vi "DisconnectionRequest.vi"(8 "AuthKey":string, 10 "Server Port":i32, 11 "Server IP":string) -> ()   [LabVIEW 2016]
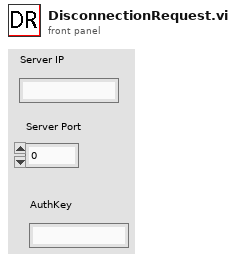
[diagram p1: front panel]
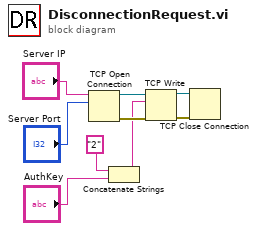
[diagram p0: block diagram]
diagram:
  n1 = TCP Open Connection(address="Server IP", remote port or service name="Server Port") -> (connection ID=w6:refnum<k5>, error out=w7:errorcluster)  [unwired: 3 in]
  n2 = Concatenate Strings("2", "AuthKey") -> (w3:string)
  n3 = TCP Write(connection ID=w6, data in=w3, error in (no error)=w7) -> (connection ID out=w2:refnum<k5>, error out=w1:errorcluster)  [unwired: 1 in, 1 out]
  n4 = TCP Close Connection(connection ID=w2, error in (no error)=w1) -> ()  [unwired: 1 in, 2 out]
